vi "Test_Complete.vi"(9 "Cycle Length":dbl=30.0 format="%#.2g", 10 "array":dbl[](array[numeric]), 11 "Heatload":bool) -> (1 "% Complete":u8(slide) scale=0.0..100.0, 2 "Time Remaining":dbl=30.0 format="%#.2g")   [LabVIEW 2014]
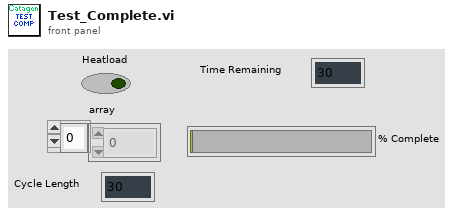
[diagram p1: front panel]
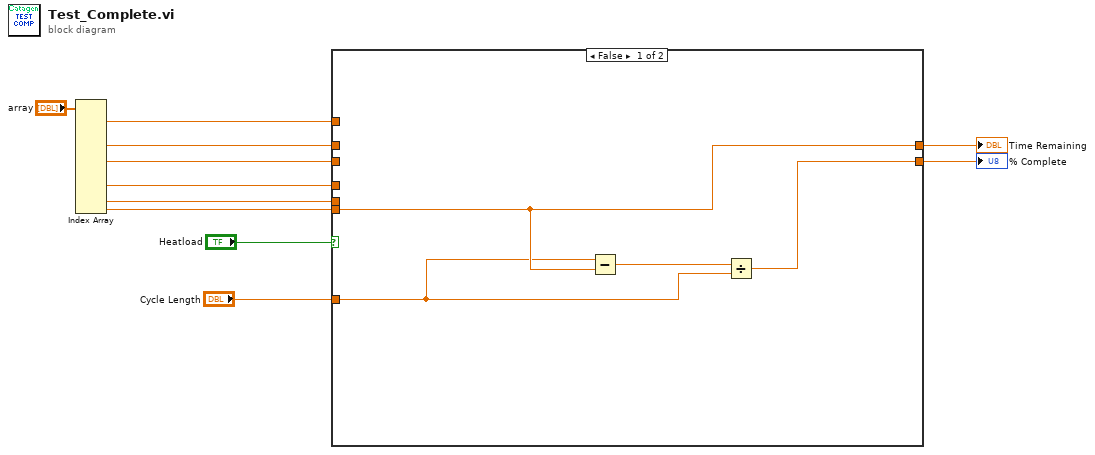
[diagram p0: block diagram]
diagram:
  n1 = Index Array(array="array") -> (element #1=w9:dbl, element #4=w7:dbl, element #6=w6:dbl, element #9=w2:dbl, element #11=w3:dbl, element #12=w1:dbl)  [unwired: 12 in, 6 out]
  n2 = case shown="False" "Heatload" {
    tunnel: "Cycle Length" -> [w13 _]
    tunnel: w9 -> [_ w22]
    tunnel: w7 -> [_ w21]
    tunnel: w6 -> [_ w20]
    tunnel: [w12 w19] -> w5
    tunnel: [w15 w18] -> w4
    tunnel: w3 -> [_ w17]
    tunnel: w2 -> [_ w16]
    tunnel: w1 -> [w15 _]
    frame False {
      n3 = Subtract(x=w13, y=w15) -> (x-y=w14:dbl)
      n4 = Divide(x=w14, y=w13) -> (x/y=w12:dbl)
    }
    frame True {
      n5 = case shown="1" w22 {
        tunnel: w21 -> [w23 _]
        tunnel: w20 -> [w24 _]
        tunnel: [w24 w26] -> w19
        tunnel: [w23 w25] -> w18
        tunnel: w17 -> [_ w26]
        tunnel: w16 -> [_ w25]
        frame 0, Default {
        }
        frame 1 {
        }
      }
    }
  }
  "% Complete" <- w5
  "Time Remaining" <- w4
